vi "create event for simulation.vi"(11 "User Event in":T1) -> (3 "User Event out":T1)   [LabVIEW 2013, in "TDMS datalogger editor node.lvclass"]
uses:
  TDMS datalogger editor node.lvclass
  <vilib>/CEF_TreeControl/Controls/EventCluster.ctl
  <vilib>/CEF_TreeControl/NISE_CEF_TreeControl.lvlib
  <vilib>/CEF_TreeControl/Node/UserEventRef.ctl
  <vilib>/CEF_TreeControl/Node/NISE_CEF_Node.lvclass
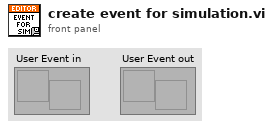
[diagram p1: front panel]
types:
  T1 = typedef "NISE_CEF_Node.lvclass/UserEventRef.ctl" = refnum<user-event>
  T2 = typedef "NISE_CEF_TreeControl.lvlib/EventCluster.ctl" = cluster{"command":string, "data":string}
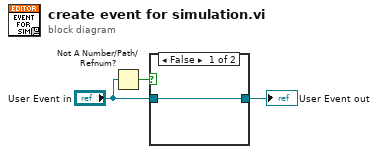
[diagram p0: block diagram]
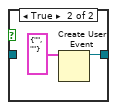
[diagram p2: hidden frame]
diagram:
  n1 = Not A Number/Path/Refnum?(number/path/refnum="User Event in") -> (NaN/Path/Refnum?=w1:bool)
  n2 = case shown="False" w1 {
    tunnel: [w4 w5] -> w2
    tunnel: "User Event in" -> [w4 _]
    frame False {
    }
    frame True {
      n3 = Create User Event(user event datatype=T2 {"command"="", "data"=""} ("event data")) -> (user event=w5:refnum<user-event>)  [unwired: 1 in, 1 out]
    }
  }
  "User Event out" <- w2
